vi "serialization tests.vi"() -> ()   [LabVIEW 2013, in "processing plugin tests.lvlib"]
uses:
  processing plugin tests.lvlib
  module/configuration/tag bus processing plugin module configuration.lvclass
  <vilib>/NI/Tag Bus Module Framework/channel/TBM channel.lvclass
panel:
  out "data":string
  out "channels equal":bool
  out "no error":errorcluster
  out "no error":errorcluster
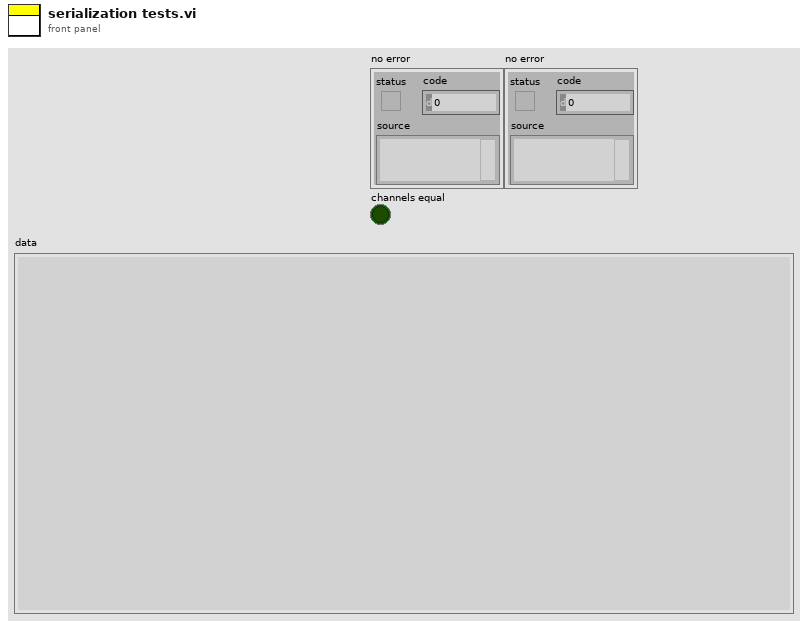
[diagram p1: front panel]
types:
  T1 = typedef "tag bus processing plugin module configuration.lvclass/processing channels.ctl" = cluster{"parameter":refnum<class "TBM channel.lvclass">, "result":refnum<class "TBM channel.lvclass">}
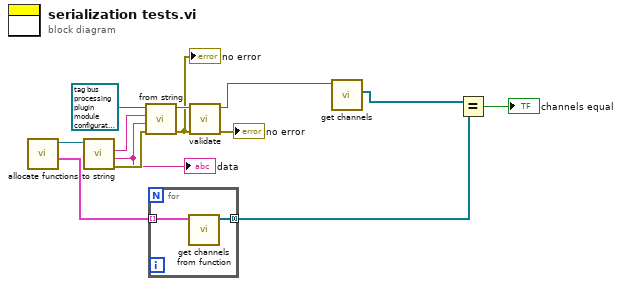
[diagram p0: block diagram]
diagram:
  n1 = call "allocate functions.vi"() -> ("functions"=w4:T1[], "tag bus processing plugin module configuration out"=w6:refnum<class "tag bus processing plugin module configuration.lvclass">)  [unwired: 9 in, 1 out]
  n2 = call-dynamic "to string.vi"("tag bus configurable plugin module configuration in"=w6) -> ("error out"=w13:errorcluster, "data"=w12:string, "version"=w11:string)  [unwired: 7 in, 1 out]
  "data" <- w12
  n3 = call-dynamic "from string.vi"("error in"=w13, "data"=w12, "version"=w11, "tag bus configurable plugin module configuration in"=refnum<class "tag bus processing plugin module configuration.lvclass"> refnum ("tag bus configurable plugin module configuration")) -> ("error out"=w8:errorcluster, "tag bus configurable plugin module configuration out"=w10:refnum<class "tag bus processing plugin module configuration.lvclass">)  [unwired: 6 in]
  "no error" <- w8
  n4 = for {
    tunnel: w4 -> [w14] mode=indexing
    tunnel: [w15] -> w3 mode=concatenating
    n5 = call "get channels from function.vi"("processing function"=w14) -> ("channels"=w15:refnum<class "TBM channel.lvclass">[])  [unwired: 10 in]
  }
  n6 = call-dynamic "validate.vi"("error in"=w8, "tag bus configurable plugin module configuration in"=w10) -> ("error out"=→"no error":errorcluster, "tag bus configurable plugin module configuration out"=w2:refnum<class "tag bus processing plugin module configuration.lvclass">)  [unwired: 8 in]
  n7 = call-dynamic "get channels.vi"("module configuration in"=w2) -> ("channels"=w1:refnum<class "TBM channel.lvclass">[])  [unwired: 9 in, 1 out]
  n8 = Equal?(x=w1, y=w3) -> (x = y?=→"channels equal":bool)
